vi "filtr_IIR.vi"(4 "Y_n-2":dbl, 6 "Y_n-1":dbl, 7 "X_n":dbl, 9 "X_n-3":dbl, 10 "X_n-2":dbl, 11 "X_n-1":dbl) -> (3 "Y_n":dbl)   [LabVIEW 2023]
doc: "Subvi sluzacy do obliczania odpowiedzi filtru IIR. Parametry filtru: N=2, M=3. Wagi a0=0,7, a1=0,3, b0=0,4, b1=0,3, b2=0,2 b3=0,1."
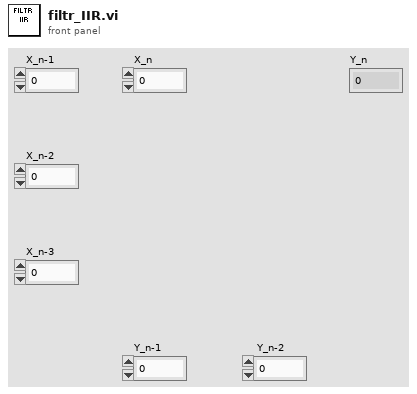
[diagram p1: front panel]
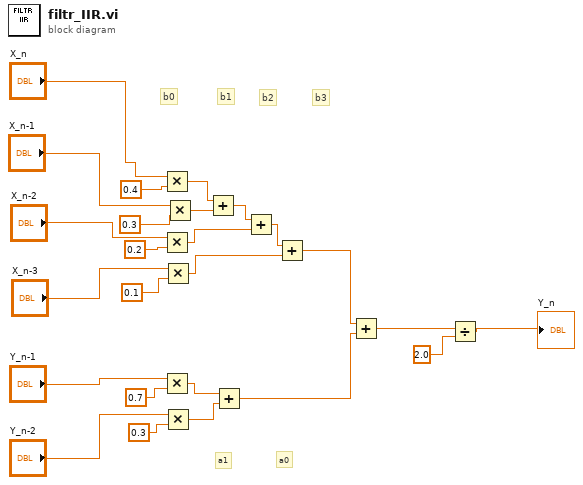
[diagram p0: block diagram]
diagram:
  # "a1"
  # "a0"
  # "b3"
  # "b2"
  # "b1"
  # "b0"
  n1 = Multiply(x="X_n", y=0.4) -> (x*y=w21:dbl)
  n2 = Multiply(x="X_n-2", y=0.2) -> (x*y=w9:dbl)
  n3 = Multiply(x="Y_n-1", y=0.7) -> (x*y=w16:dbl)
  n4 = Multiply(x="X_n-3", y=0.1) -> (x*y=w11:dbl)
  n5 = Multiply(x="Y_n-2", y=0.3) -> (x*y=w17:dbl)
  n6 = Multiply(x="X_n-1", y=0.3) -> (x*y=w7:dbl)
  n7 = Add(x=w21, y=w7) -> (x+y=w8:dbl)
  n8 = Add(x=w16, y=w17) -> (x+y=w19:dbl)
  n9 = Add(x=w8, y=w9) -> (x+y=w10:dbl)
  n10 = Add(x=w10, y=w11) -> (x+y=w18:dbl)
  n11 = Add(x=w18, y=w19) -> (x+y=w22:dbl)
  n12 = Divide(x=w22, y=2.0) -> (x/y=→"Y_n":dbl)
